vi "Determine Name of Copy.vi"(10 "All Trial Files":string[](array[string]), 11 "Trial File Path":path) -> (3 "Name of Copy":string)   [LabVIEW 2018]
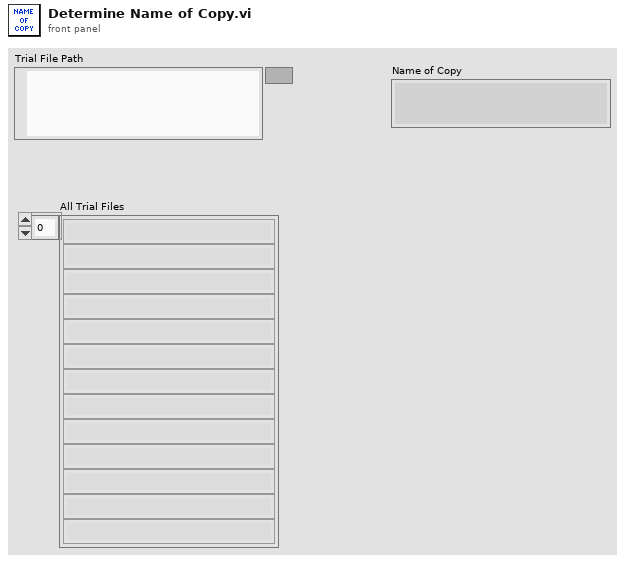
[diagram p1: front panel]
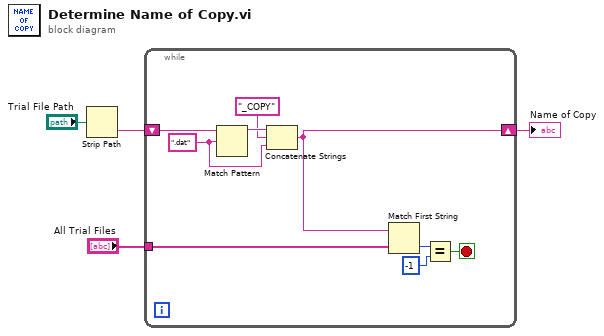
[diagram p0: block diagram]
diagram:
  n1 = Strip Path(path="Trial File Path") -> (name=w2:string)  [unwired: 1 out]
  n2 = while {
    tunnel: "All Trial Files" -> [w10]
    shift-right: [w11] -> w4
    shift-left: w2 -> [w7]
    stop <- w5 stop-if-true
    w9 = ".dat" ("regular expression")
    n3 = Match Pattern(string=w7, regular expression=w9) -> (before substring=w8:string)  [unwired: 1 in, 3 out]
    n4 = Concatenate Strings(w8, "_COPY" ("string"), w9) -> (w11:string)
    n5 = Match First String(2:w10, 3:w11) -> (0:w12:i32)  [unwired: 1 out]
    n6 = Equal?(x=w12, y=-1) -> (x = y?=w5:bool)
  }
  "Name of Copy" <- w4
